vi "UART Close.vi"(8 "Error In":errorcluster, 10 "UART Channel (0)":u8, 11 "LINX Resource":T1) -> (0 "Error Out":errorcluster, 3 "LINX Resource":T1)   [LabVIEW 2014, in "LMH-LINX.lvlib"]
doc: "Close the specified UART channel."
uses:
  <vilib>/MakerHub/LINX/LMH-LINX.lvlib
  <vilib>/MakerHub/LINX/Private/Type Defs/LINX Ref.ctl
  <vilib>/MakerHub/LINX/Private/Type Defs/Platform.ctl
  <vilib>/MakerHub/LINX/Private/Type Defs/Interface.ctl
  <vilib>/MakerHub/LINX/Private/Device/Type Defs/LINX Device Config.ctl
  <vilib>/MakerHub/LINX/Private/Device/Type Defs/TCP Config.ctl
  <vilib>/MakerHub/LINX/Private/Device/Type Defs/Channels.ctl
  <vilib>/MakerHub/LINX/Private/Type Defs/Peripheral.ctl
  <vilib>/MakerHub/LINX/Private/Type Defs/Channel FGV States.ctl
  <vilib>/MakerHub/LINX/Private/Device/Device.lvlib
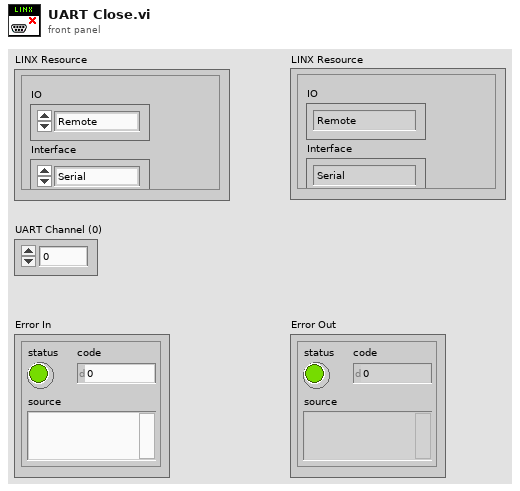
[diagram p1: front panel]
types:
  T1 = typedef "LMH-LINX.lvlib/LINX Ref.ctl" = cluster{"IO":T2, "Interface":T3, "LINX Device Config":T4}
  T2 = typedef "LMH-LINX.lvlib/Platform.ctl" = enum16{"Remote", "Local"}
  T3 = typedef "LMH-LINX.lvlib/Interface.ctl" = enum16{"Serial", "TCP"}
  T4 = typedef "LMH-LINX.lvlib/Device.lvlib/LINX Device Config.ctl" = cluster{"Interface":T3, "COM Port":refnum<visa-resource-name>, "TCP Configuration":T5, "Device Family":u8, "Device ID":u8, "Device Name":string, "TCP Ref":refnum<k5>, "Channels":T6}
  T5 = typedef "LMH-LINX.lvlib/Device.lvlib/TCP Config.ctl" = cluster{"IP Address":string, "Port":u16}
  T6 = typedef "LMH-LINX.lvlib/Channels.ctl" = cluster{"DI":u8[], "DO":u8[], "AI":u8[], "AO":u8[], "PWM":u8[], "QE":u8[], "UART":u8[], "I2C 2":u8[], "SPI":u8[], "CAN":u8[], "Servo":u8[], "AI Ref (V)":dbl, "AO Ref (V)":dbl, "AO Resolution (Bits)":u8}
  T7 = typedef "LMH-LINX.lvlib/Peripheral.ctl" = enum8{"DI", "DO", "AI", "AO", "PWM", "QE", "UART", "I2C", "SPI", "CAN", "Servo"}
  T8 = typedef "LMH-LINX.lvlib/Channel FGV States.ctl" = enum16{"Initialize", "Get", "Set"}
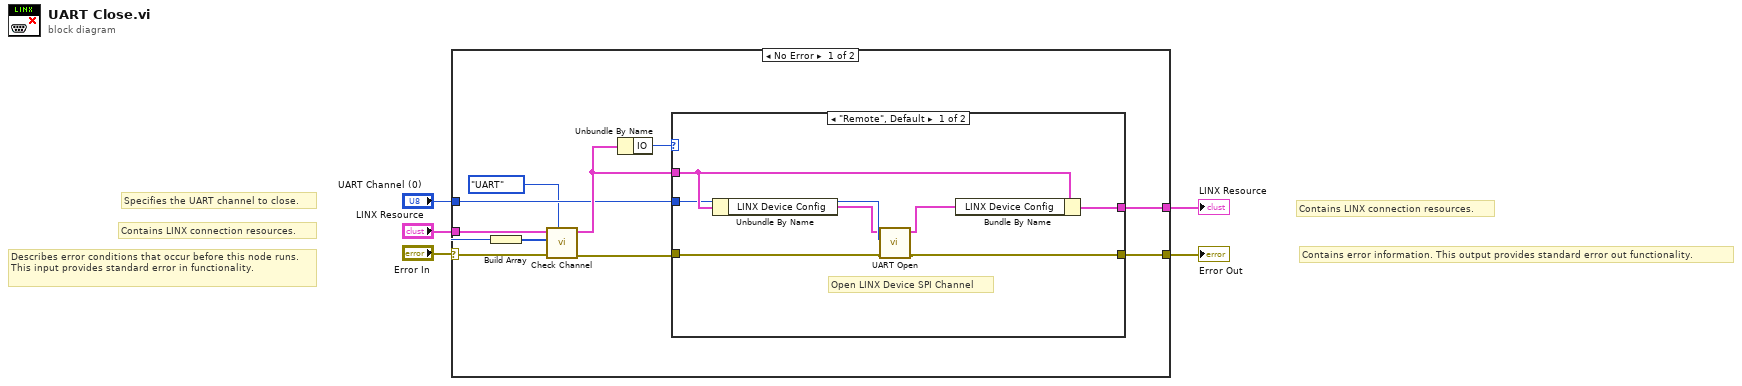
[diagram p0: block diagram]
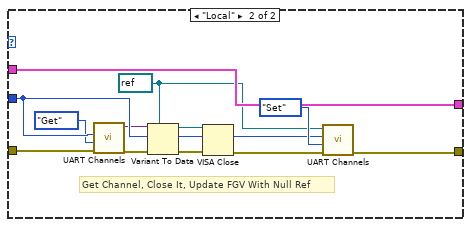
[diagram p2: hidden frame]
diagram:
  # "Specifies the UART channel to close."
  # "Contains LINX connection resources."
  # "Contains error information. This output provides standard error out functionality."
  # "Contains LINX connection resources."
  # "Describes error conditions that occur before this node runs. This input provides standard error in functionality."
  n1 = case shown="No Error" "Error In" {
    selector: "Error In" -> [w6 w36]
    tunnel: [w14 w36] -> w5
    tunnel: [w13 w35] -> w4
    tunnel: "LINX Resource" -> [w12 w35]
    tunnel: "UART Channel (0)" -> [w8 _]
    frame No Error {
      n2 = Build Array(w8) -> (w9:u8[])
      n3 = call <vilib>:"Check Channel.vi"("Peripheral"=Peripheral."UART", "Error In"=w6, "Channels"=w9, "LINX Resource"=w12) -> ("Error Out"=w10:errorcluster, "LINX Resource"=w11:T1)  [unwired: 5 in, 1 out]
      n4 = Unbundle By Name(w11) -> ("IO"=w15:T2)
      n5 = case shown="\"Remote\", Default" w15 {
        tunnel: w10 -> [w19 w31]
        tunnel: w11 -> [w22 w34]
        tunnel: [w20 w32] -> w14
        tunnel: [w21 w34] -> w13
        tunnel: w8 -> [w18 w30]
        frame "Remote", Default {
          # "Open LINX Device SPI Channel"
          n6 = Unbundle By Name(w22) -> ("LINX Device Config"=w17:T4)
          n7 = call <vilib>:"UART Open.vi"("Error In"=w19, "UART Channel"=w18, "LINX Device Config"=w17) -> ("Error Out"=w20:errorcluster, "LINX Device Config"=w16:T4)  [unwired: 6 in, 1 out]
          n8 = Bundle By Name(cluster=w22, "LINX Device Config"=w16) -> (w21:T1)
        }
        frame "Local" {
          w23 = refnum<visa-resource-name> refnum ("VISA resource name")
          # "Get Channel, Close It, Update FGV With Null Ref"
          n9 = call <vilib>:"UART Channels.vi"("Error In"=w31, "Channel State"=Channel_FGV_States."Get", "Channel Number"=w30) -> ("Error Out"=w27:errorcluster, "UART Channel"=w26:variant)  [unwired: 7 in]
          n10 = Variant To Data(error in=w27, type=w23, Variant=w26) -> (data=w25:refnum<visa-resource-name>, error out=w28:errorcluster)
          n11 = VISA Close(VISA resource name=w25, error in (no error)=w28) -> (error out=w24:errorcluster)
          n12 = call <vilib>:"UART Channels.vi"("Error In"=w24, "Channel State"=Channel_FGV_States."Set", "Channel Number"=w30, "UART Channel"=w23) -> ("Error Out"=w32:errorcluster)  [unwired: 6 in, 1 out]
        }
      }
    }
    frame Error {
    }
  }
  "Error Out" <- w5
  "LINX Resource" <- w4
